vi "Name Value Write Data.vi"(0 "Save Path":path, 7 "NameValues":string[][](array[string])) -> ()   [LabVIEW 2020]
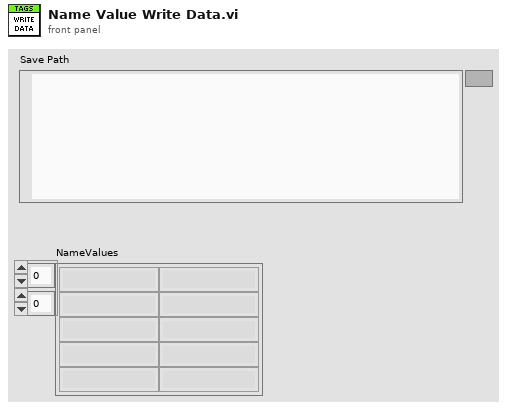
[diagram p1: front panel]
types:
  T1 = enum16{"open", "replace", "create", "open or create", "replace or create", "replace or create with confirmation"}
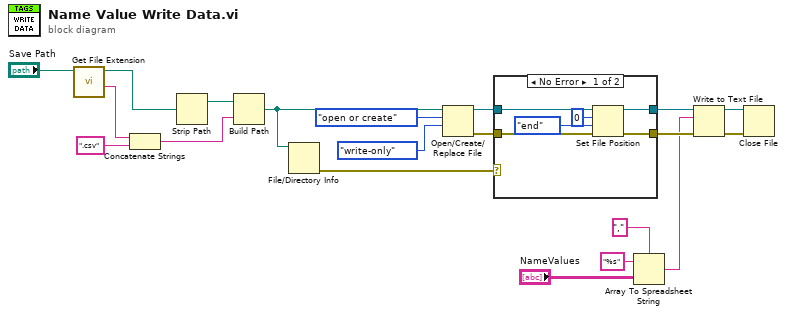
[diagram p0: block diagram]
diagram:
  n1 = call <vilib>:"Get File Extension.vi"("file"="Save Path") -> ("filename without extension"=w11:string, "dup file"=w10:path)  [unwired: 6 in, 3 out]
  n2 = Concatenate Strings(w11, ".csv" ("string")) -> (w12:string)
  n3 = Strip Path(path=w10) -> (stripped path=w9:path)  [unwired: 1 out]
  n4 = Build Path(base path=w9, name or relative path=w12) -> (appended path=w13:path)
  n5 = File/Directory Info(path=w13) -> (error out=w14:errorcluster)  [unwired: 1 in, 6 out]
  n6 = Open/Create/Replace File(file path (use dialog)=w13, operation (0:open)=T1."open or create", access (0:read/write)=enum16{"read/write", "read-only", "write-only"}."write-only") -> (refnum out=w15:refnum<file>, error out=w16:errorcluster)  [unwired: 3 in, 1 out]
  n7 = case shown="No Error" w14 {
    tunnel: w15 -> [w26 w28]
    tunnel: w16 -> [w23 w27]
    tunnel: [w22 w28] -> w17
    tunnel: [w21 w27] -> w18
    frame No Error {
      n8 = Set File Position(offset (in bytes) (0)=i64 0, refnum=w26, from (0:start)=enum16{"start", "end", "current"}."end", error in=w23) -> (refnum out=w22:refnum<file>, error out=w21:errorcluster)
    }
    frame Error {
    }
  }
  n9 = Array To Spreadsheet String(delimiter (Tab)=",", array="NameValues", 3:"%s" ("format string")) -> (spreadsheet string=w3:string)
  n10 = Write to Text File(file (use dialog)=w17, text=w3, error in=w18) -> (refnum out=w19:refnum<file>, error out=w20:errorcluster)  [unwired: 1 in, 1 out]
  n11 = Close File(refnum=w19, error in=w20) -> ()  [unwired: 2 out]
